vi "Measure.vi"(8 "error in":errorcluster, 9 "pin map context":T1, 10 "measurement configuration":T4, 11 "gRPCid in":T2) -> (0 "error out":errorcluster, 2 "measurement results":T3, 3 "gRPCid out":u64)   [LabVIEW 2021, in "Measurement Client Template.lvlib"]
doc: "Invoke the Measurement Logic and get the results"
uses:
  Measurement Client Template.lvlib
  controls/Measurement Configuration.ctl
  controls/Measurement Results.ctl
  <vilib>/gRPC/LabVIEW gRPC Library/Shared/grpcId.ctl
  <vilib>/gRPC/Generated APIs/ni/measurementlink/measurement/v2/Measurement Service Client V2/RPC Messages/ni_measurementlink_PinMapContext.ctl
  <vilib>/gRPC/Generated APIs/ni/measurementlink/measurement/v2/Measurement Service Client V2/RPC Messages/ni_measurementlink_measurement_v2_MeasureRequest.ctl
  <vilib>/gRPC/Generated APIs/ni/measurementlink/measurement/v2/Measurement Service Client V2/RPC Messages/google_protobuf_Any.ctl
  c8e7d04f-3e50-4eba-9c41-e335012f285e.vi
  233c5f21-7ff6-44c7-820f-94d9e0a33a0d.vi
  <vilib>/gRPC/LabVIEW gRPC Library/Server API/Translate Protobuf Error.vi
  <vilib>/AdvancedString/1D String Array to Delimited String.vi
  <vilib>/gRPC/LabVIEW gRPC Library/Server API/Server/Get Server DLL Path.vi
  <vilib>/gRPC/Generated APIs/ni/measurementlink/measurement/v2/Measurement Service Client V2/Measurement Service Client V2.lvlib
  <vilib>/gRPC/LabVIEW gRPC Library/grpc-lvsupport-release.lvlib
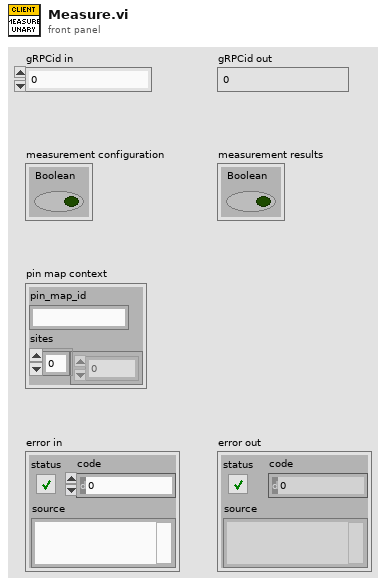
[diagram p1: front panel]
types:
  T1 = typedef "Measurement Service Client V2.lvlib/ni_measurementlink_PinMapContext.ctl" = cluster{"pin_map_id":string, "sites":i32[]}
  T2 = typedef "grpc-lvsupport-release.lvlib/grpcId.ctl" = u64
  T3 = typedef "Measurement Client Template.lvlib/Measurement Results.ctl" = cluster{"Boolean":bool}
  T4 = typedef "Measurement Client Template.lvlib/Measurement Configuration.ctl" = cluster{"Boolean":bool}
  T5 = typedef "Measurement Service Client V2.lvlib/ni_measurementlink_measurement_v2_MeasureRequest.ctl" = cluster{"configuration_parameters":T6, "pin_map_context":T1}
  T6 = typedef "Measurement Service Client V2.lvlib/google_protobuf_Any.ctl" = cluster{"type_url":string, "value":u8[]}
  T7 = typedef "grpc-lvsupport-release.lvlib/Any.ctl" = cluster{"Type Url":string, "Bytes":u8[]}
  T8 = typedef "Measurement Service Client V2.lvlib/ni_measurementlink_measurement_v2_MeasureResponse.ctl" = cluster{"outputs":T6}
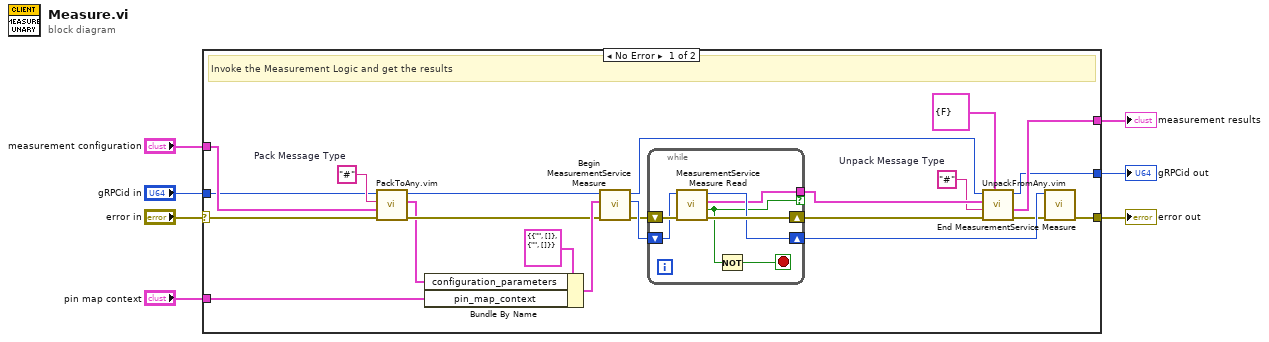
[diagram p0: block diagram]
diagram:
  n1 = case shown="No Error" "error in" {
    selector: "error in" -> [w14 w38]
    tunnel: "measurement configuration" -> [w28 _]
    tunnel: [w25 _] -> w6
    tunnel: [w21 w38] -> w5
    tunnel: "gRPCid in" -> [w13 w37]
    tunnel: [w12 w37] -> w2
    tunnel: "pin map context" -> [w9 _]
    frame No Error {
      w11 = "#"  # Unpack Message Type
      w29 = "#"  # Pack Message Type
      # "Invoke the Measurement Logic and get the results"
      n2 = call "PackToAny.vim"("error in"=w14, "Data To Pack"=w28, "Message Type"=w29, "gRPCid in"=w13) -> ("error out"=w16:errorcluster, "Any"=w8:T7, "gRPCid out"=w26:u64)  [unwired: 5 in]
      n3 = Bundle By Name(cluster=T5 {"configuration_parameters"={"type_url"="", "value"=[]}, "pin_map_context"={"pin_map_id"="", "sites"=[]}} ("Request Data"), "configuration_parameters"=w8, "pin_map_context"=w9) -> (w17:T5)
      n4 = call <vilib>:"Begin MeasurementService Measure.vi"("error in"=w16, "Request Data"=w17, "gRPC ID"=w26) -> ("error out"=w18:errorcluster, "Call Id Out"=w22:T2, "gRPC ID out"=w24:T2)  [unwired: 6 in]
      n5 = while {
        shift-right: [w35] -> w19
        shift-left: w18 -> [w36]
        shift-right: [w33] -> w23
        shift-left: w22 -> [w34]
        tunnel: [w31] -> w27 if=w30
        stop <- w32 stop-if-true
        n6 = call <vilib>:"MeasurementService Measure Read.vi"("error in"=w36, "Call ID in"=w34) -> ("error out"=w35:errorcluster, "Success"=w30:bool, "Response Data"=w31:T8, "Call ID"=w33:T2)  [unwired: 6 in]
        n7 = Not(x=w30) -> (.not. x?=w32:bool)
      }
      n8 = call "UnpackFromAny.vim"("Data Type"=T3 {"Boolean"=FALSE} ("measurement results"), "error in"=w19, "Message Type"=w11, "Any"=w27, "gRPCid in"=w24) -> ("error out"=w20:errorcluster, "Unpacked Value"=w25:T3, "gRPCid out"=w12:u64)  [unwired: 4 in]
      n9 = call <vilib>:"End MeasurementService Measure.vi"("error in"=w20, "Call ID in"=w23) -> ("error out"=w21:errorcluster)  [unwired: 8 in, 1 out]
    }
    frame Error {
      # "Pass"
    }
  }
  "measurement results" <- w6
  "gRPCid out" <- w2
  "error out" <- w5
